vi "Localized Strings.vi"() -> ()   [LabVIEW 2020, in "Add Actor.lvlib"]
uses:
  Add Actor.lvlib
panel:
  in  "This interface already exists on disk":string="This interface already exists on disk.  This operation will be skipped."
  in  "Interface for Actor":string="Interface for Actor"
  in  "You must save the library":string="You must save the library before creating actors or actor interfaces."
  in  "Error 6010":string="This target depends on multiple Actor Framework libraries.  Only one library is allowed.  You must remove the extra dependencies before proceeding."
  in  "Configure This Target":string="Configure This Target"
  in  "Actor Framework":string="Actor Framework"
  in  "Select a PPL":string="Select a packed project library"
  in  "This actor already exists on disk":string="This actor already exists on disk.  This operation will be skipped."
  in  "You must save the project":string="You must save the project before creating actors or actor interfaces."
  in  "Actor":string="Actor"
  in  "This is not an actor":string="This is not an actor. Please make another selection."
  in  "Select a parent actor":string="Select a parent actor"
  in  "Browse...":string="Browse..."
  in  "Abstract Messages for Caller":string="Abstract Messages for Caller"
  in  "Messages for this Actor":string="Messages for this Actor"
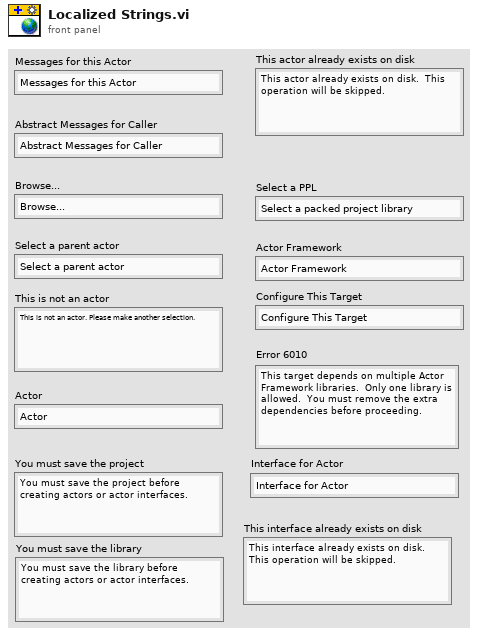
[diagram p1: front panel]
diagram:
